vi "Queue by name.vi"(4 "First Call?":bool, 5 "Queue Name":string) -> (1 "Queue":refnum<queue>)   [LabVIEW 2010]
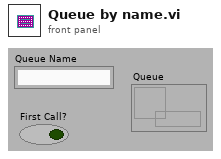
[diagram p1: front panel]
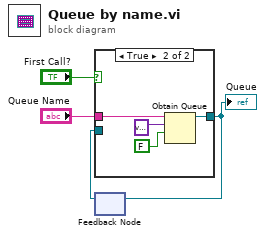
[diagram p0: block diagram]
diagram:
  n1 = feedback #1() -> (w3:refnum<queue>)  [unwired: 1 in]
  n2 = case shown="True" "First Call?" {
    tunnel: "Queue Name" -> [_ w9]
    tunnel: [w5 w6] -> w2
    tunnel: w3 -> [w5 _]
    frame False {
    }
    frame True {
      n3 = Obtain Queue(name (unnamed)=w9, element data type=variant, create if not found? (T)=FALSE) -> (queue out=w6:refnum<queue>)  [unwired: 2 in, 2 out]
    }
  }
  "Queue" <- w2
  n4 = feedback-in #1(w2) -> ()
